vi "UIinitializationCommands.vi"() -> (0 "array of cmds":T1(array[cluster]))   [LabVIEW 2017]
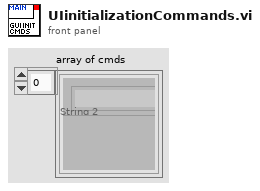
[diagram p1: front panel]
types:
  T1 = cluster{"String":string, "String 2":string, "Variant":variant}[]
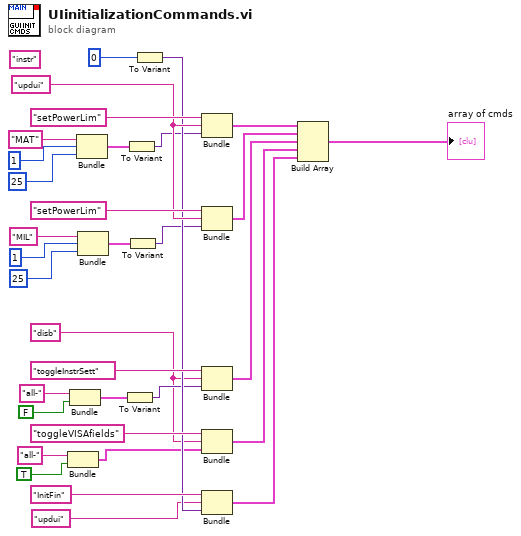
[diagram p0: block diagram]
diagram:
  w1 = "disb"
  w26 = "updui"
  (unwired) "instr"
  n1 = Bundle("all-", TRUE) -> (w2:cluster{string, bool})  [unwired: 1 in]
  n2 = Bundle("all-", FALSE) -> (w6:cluster{string, bool})  [unwired: 1 in]
  n3 = Bundle("MAT", 1, 25) -> (w19:cluster{string, i32, i32})  [unwired: 1 in]
  n4 = Bundle("MIL", 1, 25) -> (w14:cluster{string, i32, i32})  [unwired: 1 in]
  n5 = To Variant(anything=w6) -> (Variant=w9:variant)
  n6 = To Variant(anything=w19) -> (Variant=w18:variant)
  n7 = To Variant(anything=w14) -> (Variant=w12:variant)
  n8 = To Variant(anything=0) -> (Variant=w20:variant)
  n9 = Bundle("setPowerLim", w26, "Variant"=w18) -> (w31:cluster{string, string, "Variant":variant})  [unwired: 1 in]
  n10 = Bundle("setPowerLim", w26, "Variant"=w12) -> (w30:cluster{string, string, "Variant":variant})  [unwired: 1 in]
  n11 = Bundle("toggleInstrSett", w1, "Variant"=w9) -> (w25:cluster{string, string, "Variant":variant})  [unwired: 1 in]
  n12 = Bundle("toggleVISAfields", w1, w2) -> (w24:cluster{string, string, cluster{string, bool}})  [unwired: 1 in]
  n13 = Bundle("InitFin", "updui", "Variant"=w20) -> (w23:cluster{string, string, "Variant":variant})  [unwired: 1 in]
  n14 = Build Array(w31, w30, w25, w24, w23) -> (→"array of cmds":cluster{string, string, "Variant":variant}[])
